vi "sync_laser_and_camera.vi"() -> ()   [LabVIEW 2021]
doc: "This example demonstrates how to continuously generate digital pulses using a counter output."
uses:
  <vilib>/Utility/error.llb/DialogType.ctl
  <vilib>/DAQmx/create/channels.llb/DAQmx Create Channel (CO-Pulse Generation-Frequency).vi
  <vilib>/DAQmx/configure/timing.llb/DAQmx Timing (Implicit).vi
  <vilib>/DAQmx/configure/trigger.llb/DAQmx Start Trigger (Digital Edge).vi
  <resource>/objmgr/daqmx.rc
panel:
  out "Counter for Red Laser Timing":tag="Dev1/ctr0"
  out "blue duty cycle":dbl
  out "laser freq":dbl
  out "InitialRedDelay (s)":dbl
  out "Actual Duty Cycle Red":dbl
  out "Actual Frequency Red":dbl
  out "Red.Laser.Out.Term":tag
  out "Camera.Out.Term":tag
  out "Blue.Laser.Out.Term":tag caption="CO.Pulse.Term"
  in  "camera frames":dbl=2.0 min=2.0
  in  "laser pulses":dbl=1.0
  in  "Camera fps":dbl=1.0 step=1.0 format="%#.6f"
  out "Counter for Camera Timing":tag="Dev1/ctr0"
  out "Actual Duty Cycle":dbl
  out "Actual Frequency":dbl
  in  "Stop":bool
  out "Counter for Blue Laser Timing":tag="Dev1/ctr0"
  # "488 Laser Channel Settings"
  # "Camera Channel Settings"
  # "The 488 laser must be conected to PFI0 on the NI DAQ board"
  # "The camera must be conected to PFI1 on the NI DAQ board"
  # "Set the camera frames per second (fps). Make sure it is slower than the exposure time you set in the camera software"
  # "637 Laser Channel Settings"
  # "The 637 laser must be conected to PFI3 on the NI DAQ board"
  # "pulse 488 laser for"
  # "frame(s)"
  # "every"
  # "camera frames"
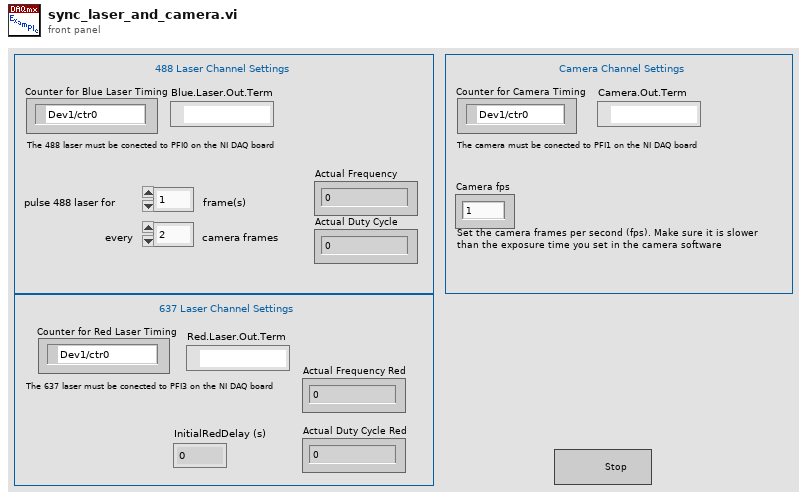
[diagram p1: front panel]
types:
  T1 = typedef "DialogType.ctl" = u16
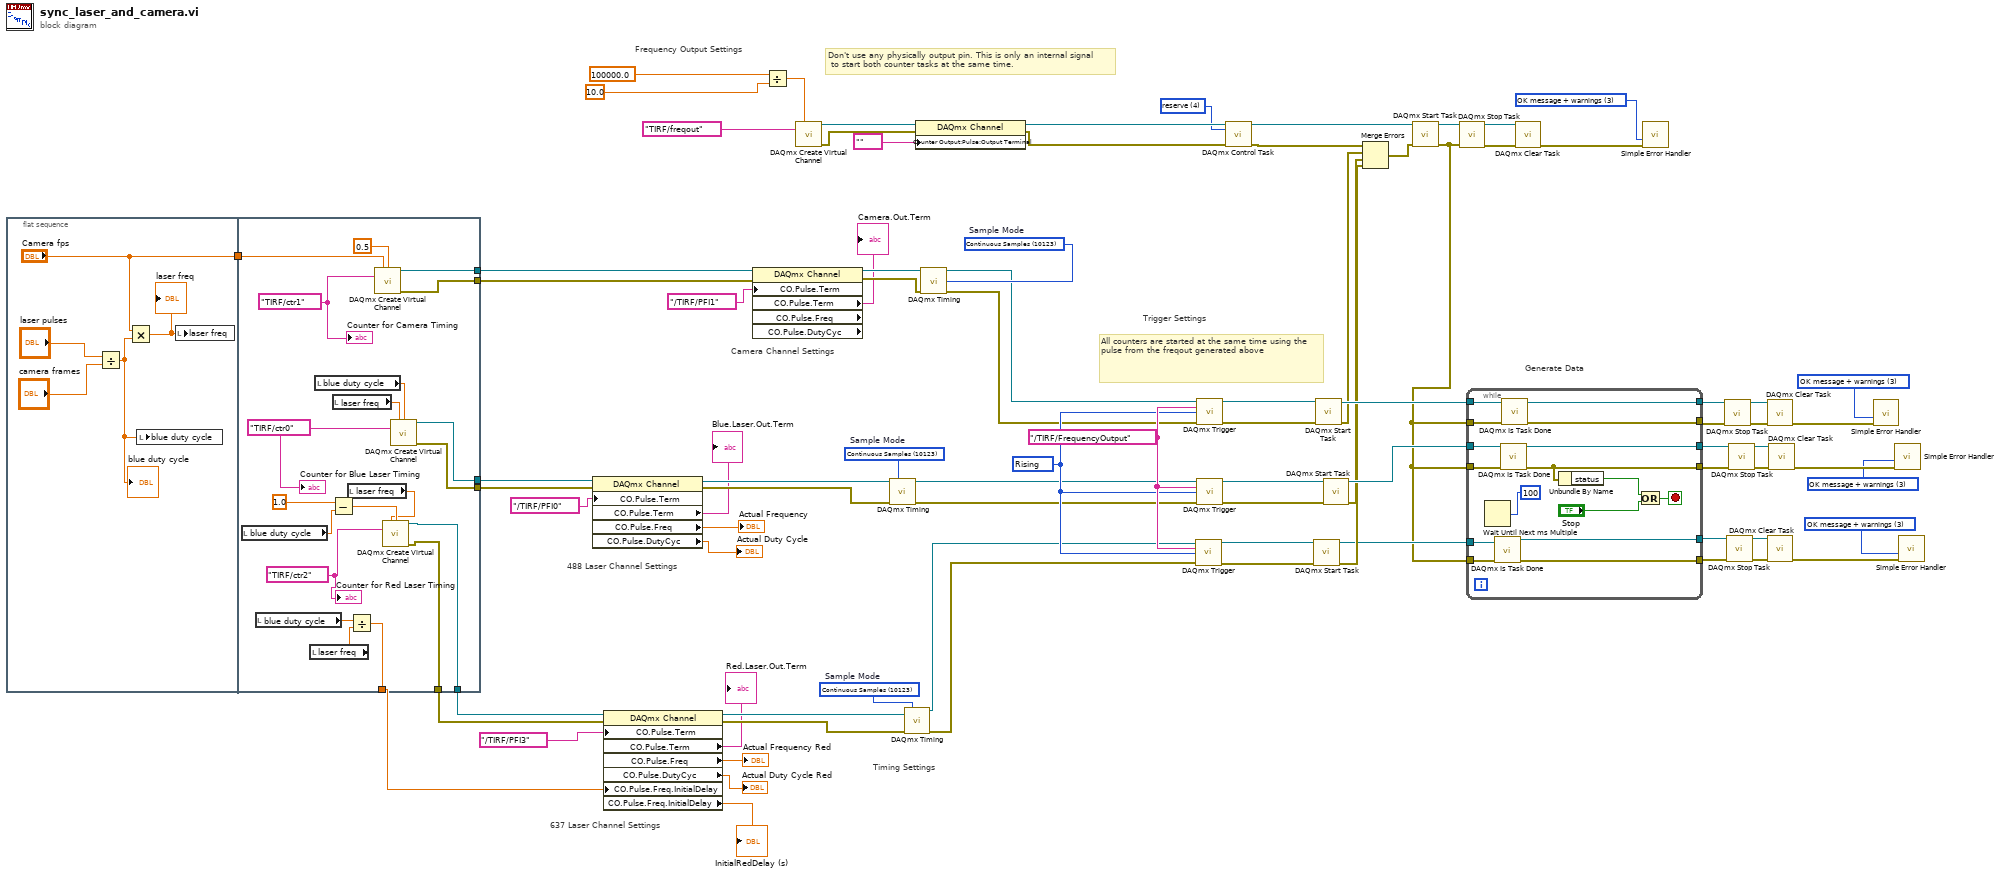
[diagram p0: block diagram]
diagram:
  w13 = 10280 items=["Rising"=10280, "Falling"=10171] ("Edge 2")
  w14 = tag "/TIRF/FrequencyOutput" ("source")
  w33 = T1 3 items=["no dialog", "OK message", "continue or stop message", "OK message + warnings", "continue/stop + warnings"] ("type of dialog (OK msg:1)")
  w40 = 10123 items=["Finite Samples"=10178, "Continuous Samples"=10123, "Hardware Timed Single Point"=12522]  # Sample Mode
  w48 = T1 3 items=["no dialog", "OK message", "continue or stop message", "OK message + warnings", "continue/stop + warnings"] ("type of dialog (OK msg:1)")
  w60 = 100000.0 items=["20MHz"=20000000.0, "10MHz"=10000000.0, "100kHz"=100000.0] ("Timebase")
  w53 = 4 items=["verify"=2, "reserve"=4, "commit"=3, "unreserve"=5, "abort"=6] ("action")
  w69 = T1 3 items=["no dialog", "OK message", "continue or stop message", "OK message + warnings", "continue/stop + warnings"] ("type of dialog (OK msg:1)")
  w75 = 10123 items=["Finite Samples"=10178, "Continuous Samples"=10123, "Hardware Timed Single Point"=12522]  # Sample Mode
  w76 = T1 3 items=["no dialog", "OK message", "continue or stop message", "OK message + warnings", "continue/stop + warnings"] ("type of dialog (OK msg:1)")
  w85 = 10123 items=["Finite Samples"=10178, "Continuous Samples"=10123, "Hardware Timed Single Point"=12522]  # Sample Mode
  # "All counters are started at the same time using the pulse from the freqout generated above"
  # "637 Laser Channel Settings"
  # "Camera Channel Settings"
  # "Frequency Output Settings"
  # "Don't use any physically output pin. This is only an internal signal\n to start both counter tasks at the same time."
  # "Generate Data"
  # "Trigger Settings"
  # "Timing Settings"
  # "488 Laser Channel Settings"
  n1 = flat-sequence {
    tunnel: ["Camera fps"] -> w24
    tunnel: w24 -> [w109]
    tunnel: [w107] -> w23
    tunnel: [w106] -> w16
    tunnel: [w103] -> w22
    tunnel: [w102] -> w21
    tunnel: [w96] -> w19
    tunnel: [w95] -> w18
    tunnel: [w92] -> w17
    frame #0 {
      n2 = Divide(x="laser pulses", y="camera frames") -> (x/y=w86:dbl)
      "blue duty cycle" <- w86
      n3 = Multiply(x="Camera fps", y=w86) -> (x*y=w87:dbl)
      "laser freq" <- w87
      n4 = local write "blue duty cycle"(w86) -> ()
      n5 = local write "laser freq"(w87) -> ()
    }
    frame #1 {
      w91 = tag "TIRF/ctr2" ("counter")
      w104 = tag "TIRF/ctr0" ("Counter")
      w110 = tag "TIRF/ctr1" ("Counter 2")
      n6 = local read "blue duty cycle"() -> (w99:dbl)
      n7 = local read "blue duty cycle"() -> (w93:dbl)
      n8 = local read "laser freq"() -> (w94:dbl)
      n9 = local read "blue duty cycle"() -> (w101:dbl)
      n10 = Subtract(x=1.0, y=w99) -> (x-y=w98:dbl)
      n11 = local read "laser freq"() -> (w105:dbl)
      n12 = local read "laser freq"() -> (w97:dbl)
      n13 = Divide(x=w93, y=w94) -> (x/y=w92:dbl)
      n14 = call-poly <vilib>:"DAQmx Create Virtual Channel.vi"("frequency"=w109, "duty cycle"=0.5, "counter"=w110) -> ("task out"=w107:refnum<k21>, "error out"=w106:errorcluster)  [unwired: 11 in]
      n15 = call-poly <vilib>:"DAQmx Create Virtual Channel.vi"("frequency"=w97, "duty cycle"=w98, "counter"=w91) -> ("task out"=w102:refnum<k21>, "error out"=w95:errorcluster)  [unwired: 11 in]
      n16 = call-poly <vilib>:"DAQmx Create Virtual Channel.vi"("frequency"=w105, "duty cycle"=w101, "counter"=w104) -> ("task out"=w103:refnum<k21>, "error out"=w96:errorcluster)  [unwired: 11 in]
      "Counter for Camera Timing" <- w110
      "Counter for Blue Laser Timing" <- w104
      "Counter for Red Laser Timing" <- w91
    }
  }
  n17 = property class="DAQmx Channel"(reference=w22, error in=w19, "CO.Pulse.Term"=tag "/TIRF/PFI0" ("Output Terminal")) -> (reference out=w81:refnum<k21>, error out=w82:errorcluster, "CO.Pulse.Term"=→"Blue.Laser.Out.Term":tag, "CO.Pulse.Freq"=→"Actual Frequency":dbl, "CO.Pulse.DutyCyc"=→"Actual Duty Cycle":dbl)
  n18 = property class="DAQmx Channel"(reference=w21, error in=w18, "CO.Pulse.Term"=tag "/TIRF/PFI3", "CO.Pulse.Freq.InitialDelay"=w17) -> (reference out=w38:refnum<k21>, error out=w39:errorcluster, "CO.Pulse.Term"=→"Red.Laser.Out.Term":tag, "CO.Pulse.Freq"=→"Actual Frequency Red":dbl, "CO.Pulse.DutyCyc"=→"Actual Duty Cycle Red":dbl, "CO.Pulse.Freq.InitialDelay"=→"InitialRedDelay (s)":dbl)
  n19 = property class="DAQmx Channel" props=["CO.Pulse.Term", "CO.Pulse.Term", "CO.Pulse.Freq", "CO.Pulse.DutyCyc"](reference=w23, error in=w16, "CO.Pulse.Term"=tag "/TIRF/PFI1") -> (reference out=w74:refnum<k21>, error out=w73:errorcluster, "CO.Pulse.Term"=→"Camera.Out.Term":tag)  [unwired: 2 out]
  n20 = Divide(x=w60, y=10.0 ("Divisor (1-16)")) -> (x/y=w52:dbl)
  n21 = call-poly <vilib>:"DAQmx Create Virtual Channel.vi"("frequency"=w52, "counter"=tag "TIRF/freqout") -> ("task out"=w57:refnum<k21>, "error out"=w56:errorcluster)  [unwired: 12 in]
  n22 = call-poly <vilib>:"DAQmx Timing.vi"("task/channels in"=w81, "sample mode"=w85, "error in"=w82) -> ("task out"=w9:refnum<k21>, "error out"=w10:errorcluster)  [unwired: 11 in]
  n23 = call-poly <vilib>:"DAQmx Timing.vi"("task/channels in"=w38, "sample mode"=w40, "error in"=w39) -> ("task out"=w8:refnum<k21>, "error out"=w7:errorcluster)  [unwired: 11 in]
  n24 = property class="DAQmx Channel"(reference=w57, error in=w56, "Counter Output:Pulse:Output Terminal"=tag "" ("CO.Pulse.Term")) -> (reference out=w55:refnum<k21>, error out=w54:errorcluster)
  n25 = call-poly <vilib>:"DAQmx Timing.vi"("task/channels in"=w74, "sample mode"=w75, "error in"=w73) -> ("task out"=w12:refnum<k21>, "error out"=w11:errorcluster)  [unwired: 11 in]
  n26 = call-poly <vilib>:"DAQmx Trigger.vi"("task/channels in"=w8, "source"=w14, "edge"=w13, "error in"=w7) -> ("task out"=w2:refnum<k21>, "error out"=w1:errorcluster)  [unwired: 10 in]
  n27 = call-poly <vilib>:"DAQmx Trigger.vi"("task/channels in"=w9, "source"=w14, "edge"=w13, "error in"=w10) -> ("task out"=w4:refnum<k21>, "error out"=w3:errorcluster)  [unwired: 10 in]
  n28 = call-poly <vilib>:"DAQmx Trigger.vi"("task/channels in"=w12, "source"=w14, "edge"=w13, "error in"=w11) -> ("task out"=w6:refnum<k21>, "error out"=w5:errorcluster)  [unwired: 10 in]
  n29 = call <vilib>:"DAQmx Control Task.vi"("task/channels in"=w55, "action"=w53, "error in"=w54) -> ("task out"=w50:refnum<k21>, "error out"=w44:errorcluster)  [unwired: 11 in]
  n30 = call <vilib>:"DAQmx Start Task.vi"("task/channels in"=w2, "error in"=w1) -> ("task out"=w32:refnum<k21>, "error out"=w37:errorcluster)  [unwired: 12 in]
  n31 = call <vilib>:"DAQmx Start Task.vi"("task/channels in"=w6, "error in"=w5) -> ("task out"=w68:refnum<k21>, "error out"=w42:errorcluster)  [unwired: 12 in]
  n32 = call <vilib>:"DAQmx Start Task.vi"("task/channels in"=w4, "error in"=w3) -> ("task out"=w84:refnum<k21>, "error out"=w41:errorcluster)  [unwired: 12 in]
  n33 = Merge Errors(w44, w42, w41, w37) -> (w43:errorcluster)
  n34 = call <vilib>:"DAQmx Start Task.vi"("task/channels in"=w50, "error in"=w43) -> ("task out"=w45:refnum<k21>, "error out"=w29:errorcluster)  [unwired: 12 in]
  n35 = call <vilib>:"DAQmx Stop Task.vi"("task/channels in"=w45, "error in"=w29) -> ("task out"=w47:refnum<k21>, "error out"=w46:errorcluster)  [unwired: 12 in]
  n36 = while {
    tunnel: w84 -> [w126]
    tunnel: [w123] -> w77
    tunnel: [w124] -> w78
    tunnel: w68 -> [w119]
    tunnel: w29 -> [w118]
    tunnel: [w117] -> w67
    tunnel: [w116] -> w66
    tunnel: w29 -> [w115]
    tunnel: w32 -> [w114]
    tunnel: [w113] -> w31
    tunnel: [w112] -> w30
    tunnel: w29 -> [w111]
    stop <- w125 stop-if-true
    n37 = Wait Until Next ms Multiple(millisecond multiple=u32 100) -> ()  [unwired: 1 out]
    n38 = call <vilib>:"DAQmx Is Task Done.vi"("task/channels in"=w114, "error in"=w111) -> ("task out"=w113:refnum<k21>, "error out"=w112:errorcluster)  [unwired: 11 in, 1 out]
    n39 = call <vilib>:"DAQmx Is Task Done.vi"("task/channels in"=w126, "error in"=w115) -> ("task out"=w124:refnum<k21>, "error out"=w123:errorcluster)  [unwired: 11 in, 1 out]
    n40 = call <vilib>:"DAQmx Is Task Done.vi"("task/channels in"=w119, "error in"=w118) -> ("task out"=w117:refnum<k21>, "error out"=w116:errorcluster)  [unwired: 11 in, 1 out]
    n41 = Unbundle By Name(w123) -> ("status"=w122:bool)
    n42 = Or(x=w122, y="Stop") -> (x .or. y?=w125:bool)
  }
  n43 = call <vilib>:"DAQmx Clear Task.vi"("task in"=w47, "error in"=w46) -> ("error out"=w49:errorcluster)  [unwired: 13 in]
  n44 = call <vilib>:"Simple Error Handler.vi"("type of dialog (OK msg:1)"=w48, "error in (no error)"=w49) -> ()  [unwired: 3 in, 5 out]
  n45 = call <vilib>:"DAQmx Stop Task.vi"("task/channels in"=w67, "error in"=w66) -> ("task out"=w71:refnum<k21>, "error out"=w70:errorcluster)  [unwired: 12 in]
  n46 = call <vilib>:"DAQmx Stop Task.vi"("task/channels in"=w31, "error in"=w30) -> ("task out"=w35:refnum<k21>, "error out"=w34:errorcluster)  [unwired: 12 in]
  n47 = call <vilib>:"DAQmx Stop Task.vi"("task/channels in"=w78, "error in"=w77) -> ("task out"=w80:refnum<k21>, "error out"=w79:errorcluster)  [unwired: 12 in]
  n48 = call <vilib>:"DAQmx Clear Task.vi"("task in"=w71, "error in"=w70) -> ("error out"=w72:errorcluster)  [unwired: 13 in]
  n49 = call <vilib>:"DAQmx Clear Task.vi"("task in"=w35, "error in"=w34) -> ("error out"=w36:errorcluster)  [unwired: 13 in]
  n50 = call <vilib>:"DAQmx Clear Task.vi"("task in"=w80, "error in"=w79) -> ("error out"=w83:errorcluster)  [unwired: 13 in]
  n51 = call <vilib>:"Simple Error Handler.vi"("type of dialog (OK msg:1)"=w69, "error in (no error)"=w72) -> ()  [unwired: 3 in, 5 out]
  n52 = call <vilib>:"Simple Error Handler.vi"("type of dialog (OK msg:1)"=w76, "error in (no error)"=w83) -> ()  [unwired: 3 in, 5 out]
  n53 = call <vilib>:"Simple Error Handler.vi"("type of dialog (OK msg:1)"=w33, "error in (no error)"=w36) -> ()  [unwired: 3 in, 5 out]
